vi "Hardware Device Get Info.vi"(8 "error in":errorcluster, 11 "NI Digital Output in":refnum<class "NI Digital Output.lvclass">) -> (0 "error out":errorcluster, 3 "NI Digital Output out":refnum<class "NI Digital Output.lvclass">)   [LabVIEW 2023, in "HardwareAbstractionLayer_LVOOP.lvlib" / "NI Digital Output.lvclass"]
doc: "This VI Device Physical Channel Read"
uses:
  NI Digital Output.lvclass
  NI Digital Output.lvclass/NI Digital Output.ctl
  <resource>/objmgr/daqmx.rc
  Teststand/Teststand.lvclass
panel:
  out "DO.PhysicalChans":tag[](array[tag])
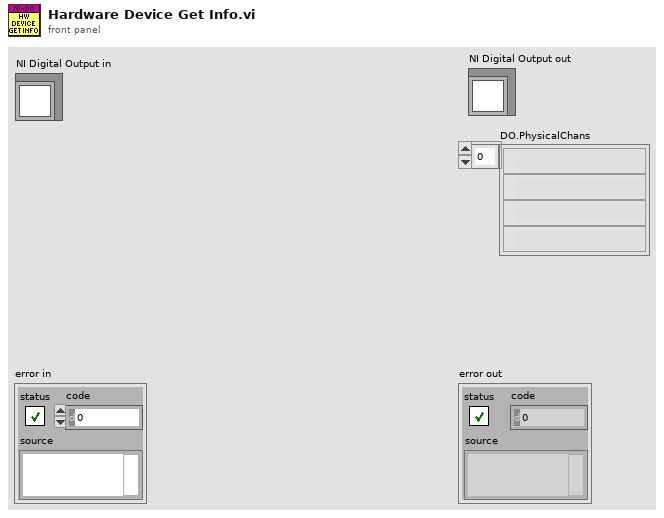
[diagram p1: front panel]
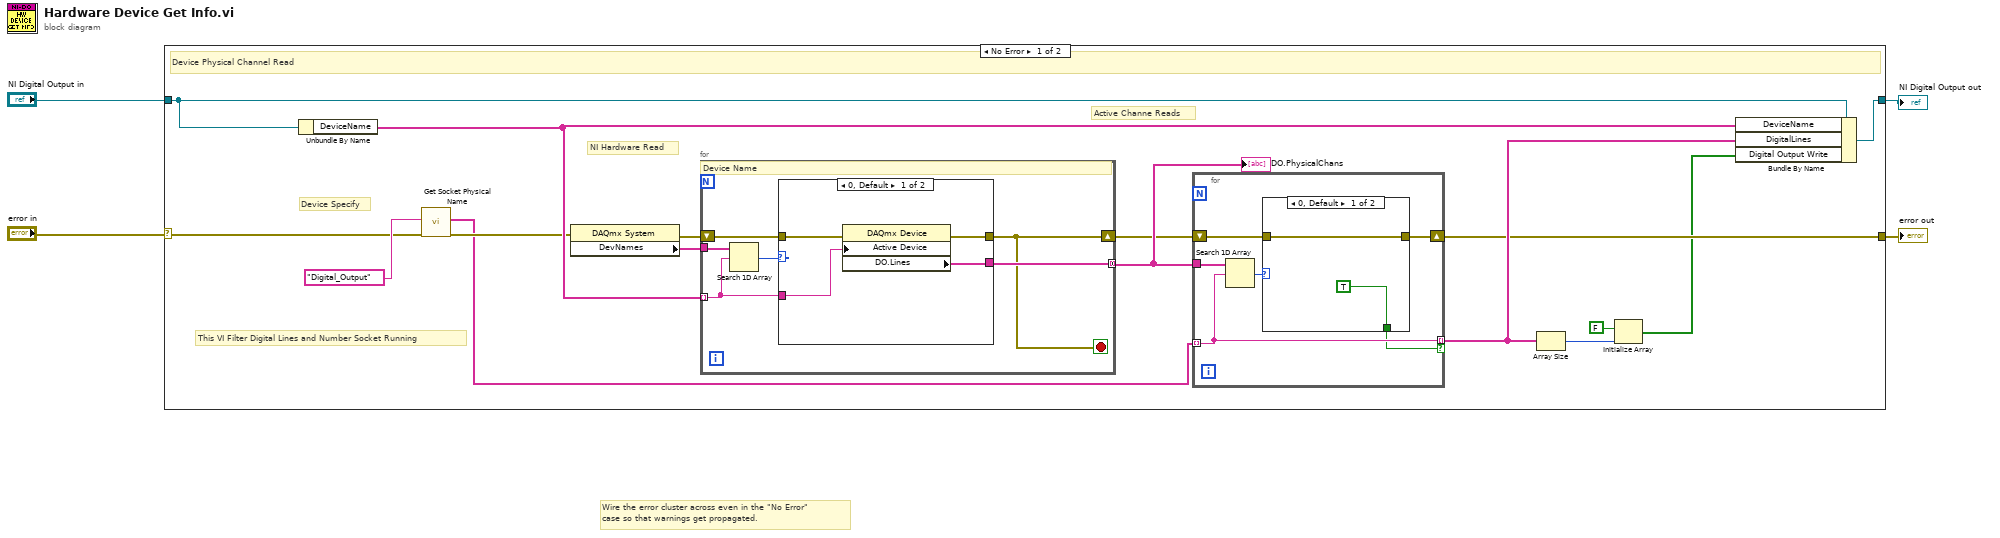
[diagram p0: block diagram]
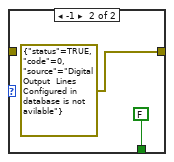
[diagram p2: hidden frame]
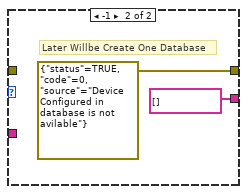
[diagram p3: hidden frame]
diagram:
  # "Wire the error cluster across even in the \"No Error\"\ncase so that warnings get propagated."
  n1 = case shown="No Error" "error in" {
    selector: "error in" -> [w7 w44]
    tunnel: [w10 w44] -> w3
    tunnel: [w15 w43] -> w1
    tunnel: "NI Digital Output in" -> [w14 w43]
    frame No Error {
      # "This VI Filter Digital Lines and Number Socket Running"
      # "Active Channe Reads"
      # "Device Specify"
      # "NI Hardware Read"
      # "Device Physical Channel Read"
      n2 = Unbundle By Name(w14) -> ("DeviceName"=w20:tag[])
      n3 = call "Get Socket Physical Name.vi"("error In"=w7, "ChannelType"="Digital_Output") -> ("error out"=w6:errorcluster, "Physical Channel"=w5:tag[])  [unwired: 7 in, 1 out]
      n4 = property class="DAQmx System"(error in=w6) -> (error out=w18:errorcluster, "DevNames"=w19:tag[])  [unwired: 1 in, 1 out]
      n5 = for {
        tunnel: w20 -> [w33] mode=indexing
        tunnel: w19 -> [w34]
        tunnel: [w32] -> w17 mode=concatenating
        shift-right: [w31] -> w16
        shift-left: w18 -> [w35]
        stop <- w31 stop-if-true
        # "Device Name"
        n6 = Search 1D Array(1D array=w34, element=w33) -> (index of element=w36:i32)  [unwired: 1 in]
        n7 = case shown="0, Default" w36 {
          tunnel: w35 -> [w38 _]
          tunnel: [w37 errorcluster {"status"=TRUE, "code"=0, "source"="Device  Configured in database is not avilable"} ("error out")] -> w31
          tunnel: w33 -> [w40 _]
          tunnel: [w39 tag[] [] ("AI.PhysicalChans")] -> w32
          frame 0, Default {
            n8 = property class="DAQmx Device"(error in=w38, "Active Device"=w40) -> (error out=w37:errorcluster, "DO.Lines"=w39:tag[])  [unwired: 1 in, 1 out]
          }
          frame -1 {
            # "Later Willbe Create One Database"
          }
        }
      }
      "DO.PhysicalChans" <- w17
      n9 = for {
        tunnel: w17 -> [w26]
        tunnel: w5 -> [w22] mode=indexing
        shift-right: [w23] -> w10
        shift-left: w16 -> [w24]
        tunnel: [w22] -> w13 mode=indexing if=w21
        n10 = Search 1D Array(1D array=w26, element=w22) -> (index of element=w25:i32)  [unwired: 1 in]
        n11 = case shown="0, Default" w25 {
          tunnel: w24 -> [w28 _]
          tunnel: [w28 errorcluster {"status"=TRUE, "code"=0, "source"="Digital Output  Lines Configured in database is not avilable"} ("error out")] -> w23
          tunnel: [TRUE FALSE] -> w21
          frame 0, Default {
          }
          frame -1 {
          }
        }
      }
      n12 = Array Size(array=w13) -> (size(s)=w12:i32)
      n13 = Initialize Array(FALSE, w12) -> (w9:bool[])
      n14 = Bundle By Name(cluster=w14, "DeviceName"=w20, "DigitalLines"=w13, "Digital Output Write"=w9) -> (w15:refnum<class "NI Digital Output.lvclass">)
    }
    frame Error {
    }
  }
  "error out" <- w3
  "NI Digital Output out" <- w1
